vi "Init Client Data.vi"(8 "error in (no error)":errorcluster, 10 "Authentication":T1, 11 "Server Init Data":T2 {"Server Status" format="%.0x"; "Server Languague" format="%.0x"; "Server Capabilities" format="%.0x"}) -> (0 "error out":errorcluster, 3 "TCPIP Data":u8[](array[numeric]))   [LabVIEW 2014, in "hse-db.lvlib" / "MySQL (TCP).lvlib"]
uses:
  MySQL (TCP).lvlib
  Controls/Server Init Data.ctl
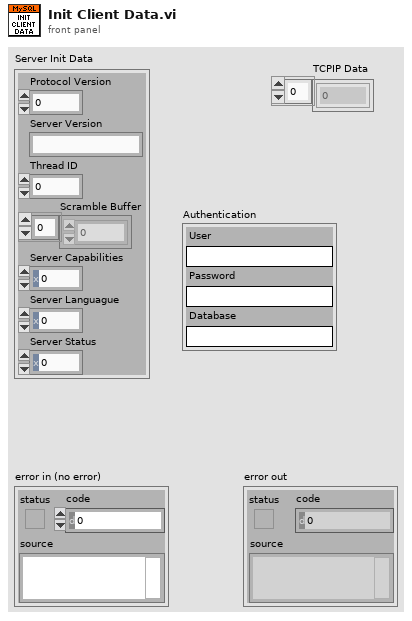
[diagram p1: front panel]
types:
  T1 = cluster{"User":string, "Password":string, "Database":string}
  T2 = typedef "hse-db.lvlib/MySQL (TCP).lvlib/Server Init Data.ctl" = cluster{"Protocol Version":u8, "Server Version":string, "Thread ID":u32, "Scramble Buffer":u8[], "Server Capabilities":u16, "Server Languague":u8, "Server Status":u16}
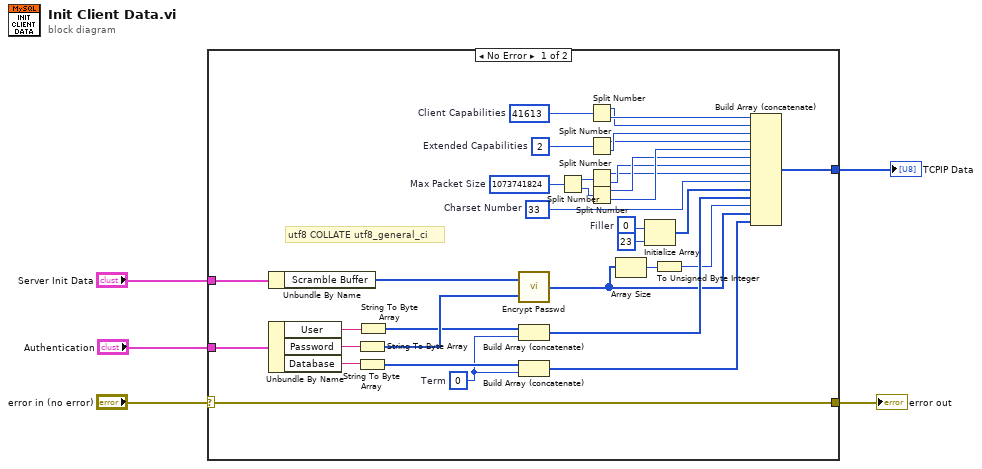
[diagram p0: block diagram]
diagram:
  n1 = case shown="No Error" "error in (no error)" {
    selector: "error in (no error)" -> [w39 w40]
    tunnel: [w39 w40] -> w5
    tunnel: "Server Init Data" -> [w38 _]
    tunnel: [w20 _] -> w2
    tunnel: "Authentication" -> [w23 _]
    frame No Error {
      w6 = u8 0  # Term
      w15 = u8 0  # Filler
      w33 = u16 2  # Extended Capabilities
      w37 = u16 41613  # Client Capabilities
      w24 = u8 33  # Charset Number
      w34 = u32 1073741824  # Max Packet Size
      # "utf8 COLLATE utf8_general_ci"
      n2 = Unbundle By Name(w38) -> ("Scramble Buffer"=w18:u8[])
      n3 = Unbundle By Name(w23) -> ("User"=w22:string, "Password"=w19:string, "Database"=w21:string)
      n4 = String To Byte Array(string=w19) -> (unsigned byte array=w17:u8[])
      n5 = String To Byte Array(string=w21) -> (unsigned byte array=w11:u8[])
      n6 = String To Byte Array(string=w22) -> (unsigned byte array=w13:u8[])
      n7 = call "Encrypt Passwd.vi"("Data"=w17, "Scramble"=w18) -> ("SHA1 Data"=w9:u8[])
      n8 = Build Array (concatenate)(w13, w6) -> (w12:u8[])
      n9 = Build Array (concatenate)(w11, w6) -> (w10:u8[])
      n10 = Split Number(x=w34) -> (hi(x)=w35:u16, lo(x)=w36:u16)
      n11 = Split Number(x=w37) -> (hi(x)=w31:u8, lo(x)=w32:u8)
      n12 = Split Number(x=w33) -> (hi(x)=w29:u8, lo(x)=w30:u8)
      n13 = Split Number(x=w35) -> (hi(x)=w25:u8, lo(x)=w26:u8)
      n14 = Split Number(x=w36) -> (hi(x)=w27:u8, lo(x)=w28:u8)
      n15 = Array Size(array=w9) -> (size(s)=w8:i32)
      n16 = Initialize Array(w15, 23 ("dimension size")) -> (w14:u8[])
      n17 = To Unsigned Byte Integer(number=w8) -> (unsigned 8bit integer=w7:u8)
      n18 = Build Array (concatenate)(w32, w31, w30, w29, w28, w27, w26, w25, w24, w14, w12, w7, w9, w10) -> (w20:u8[])
    }
    frame Error {
    }
  }
  "error out" <- w5
  "TCPIP Data" <- w2
